vi "SeCrTs-RD Modified.vi"() -> ()   [LabVIEW 2022 SP3]
doc: "Datalog Redundant software"
uses:
  SeCrTS-Display And Datalog/Source Code/Control/SeCrTs-Enum.ctl
  Source Code/Globals/SeCrTs-RD globals.vi
panel:
  out "Logging?":bool
  out "Connected?":bool
  in  "Exit":bool
  out "Log Period(Min)":dbl
  out "Log type":bool
  in  "IP Address":string="169.254.222.222"
  out "error out":errorcluster
  # "DATALOG REDUNDANT SOFTWARE"
  # "VERSION           : V1.2\nRELEASE DATE : 23/09/2024"
  # "Periodical log"
  # "Continuous log"
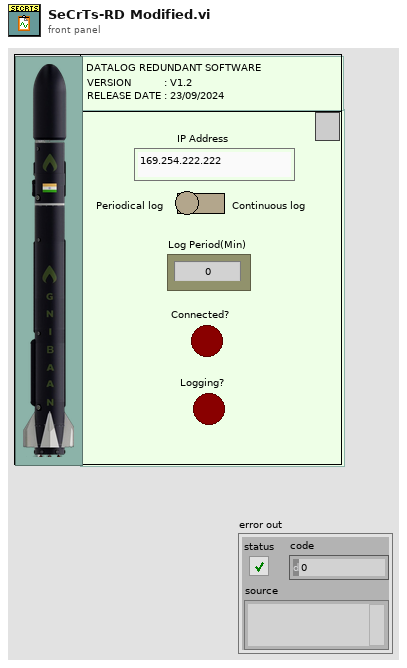
[diagram p1: front panel]
types:
  T1 = typedef "SeCrTs-Enum.ctl" = enum16{"Initialize", "Poll", "Establish ref", "Read", "Close", "Exit"}
  T2 = cluster{"Config":refnum<k21>, "log":refnum<k21>, "Log name":refnum<k21>, "C/NC":refnum<k21>, "Log time":refnum<k21>}
  T3 = enum8{"Enabled", "Disabled", "Disabled and Grayed Out"}
  T4 = cluster{"AO config":cluster{"Channel_Name":string, "Channel_Number":string, "Default_Value":dbl, "Units":string}[], "AI config":cluster{"Channel_Name":string, "Channel_Number":string, "Pre_Scale_min":dbl, "Pre_Scale_max":dbl, "Sensor_min":dbl, "Sensor_max":dbl, "Units":string}[], "DI config":cluster{"Channel_Name":string, "Channel_Number":string, "Default_Value":bool, "DI invert?":bool}[], "DO config":cluster{"Channel_Name":string, "Channel_Number":string, "Default_Value":bool, "DO invert?":bool}[], "TC config":cluster{"Channel_Name":string, "Channel_Number":string, "Pre_Scale_min":dbl, "Pre_Scale_max":dbl, "units":i32, " type":i32}[], "ACC config":cluster{"Channel_Name":string, "Channel_Number":string, "Pre_Scale_min":dbl, "Pre_Scale_max":dbl, "Terminal configuration":i32, "Sensitivity":dbl, "Sensitivity units":i32}[], "SG config":cluster{"Channel_Name":string, "Channel_Number":string, "Pre_Scale_min":dbl, "Pre_Scale_max":dbl}[], "Strain Gauge Settings":cluster{"poisson ratio":dbl, "nominal gage resistance":dbl, "gage factor":dbl}, "Bridge Settings":cluster{"voltage excitation value":dbl, "voltage excitation source":i32, "initial bridge voltage":dbl, "lead wire resistance":dbl, "strain configuration":i32}, "Sample Rate":cluster{"AI Sample Rate":dbl[], "AO Sample Rate":dbl[], "DI Sample Rate":dbl[], "TC Sample Rate":dbl[], "DO Sample Rate":dbl[], "SG Sample Rate":dbl[], "ACC Sample Rate":dbl[]}}
  T5 = enum32{"invalid app kind", "Development System", "Run Time System", "Student Edition", "Embedded LabVIEW", "Evaluation", "Custom"}
  T6 = cluster{"Datalog path":path, "Configuration path":path, "Signal list path":path, "Sub vi's":path, "Authentication":path}
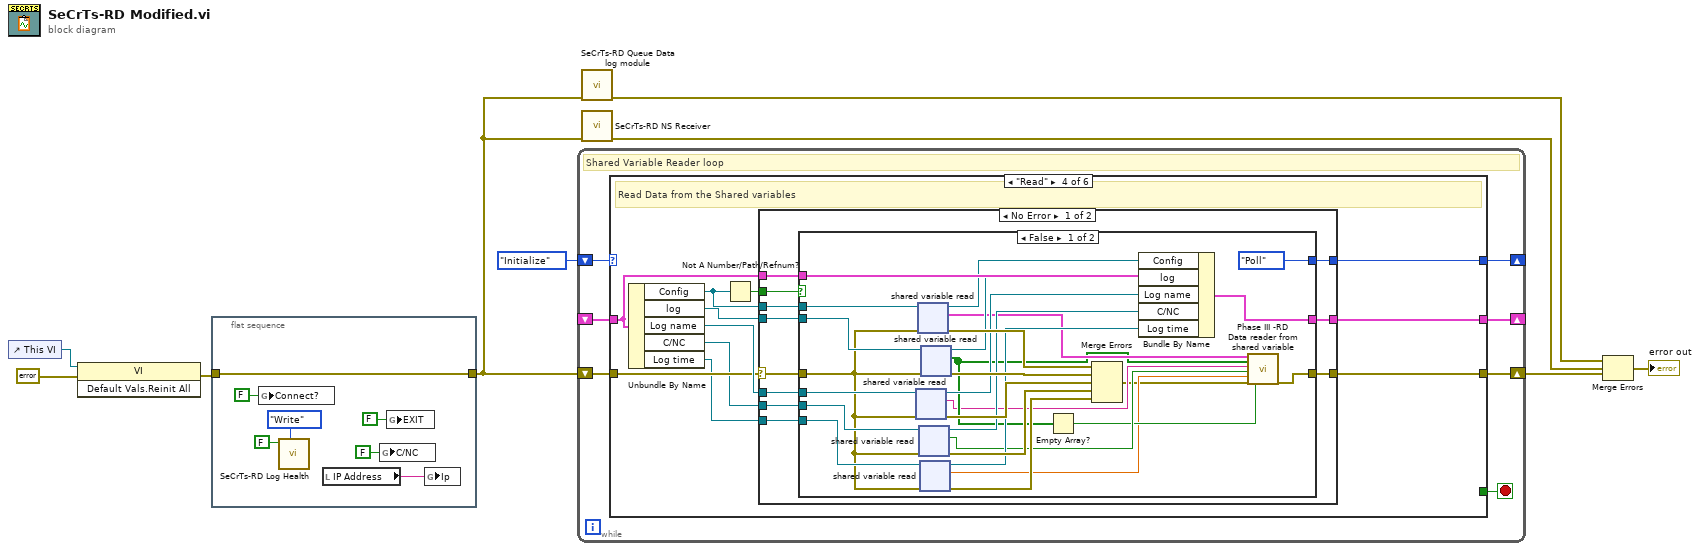
[diagram p0: block diagram]
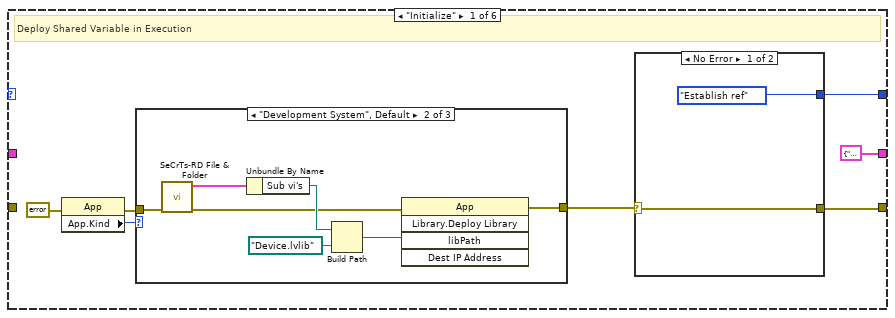
[diagram p2: hidden frame]
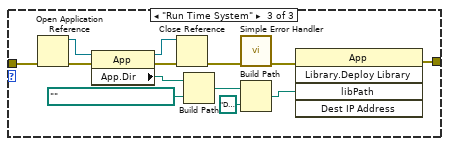
[diagram p4: hidden frame]
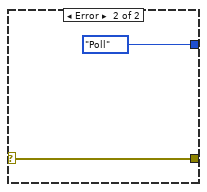
[diagram p5: hidden frame]
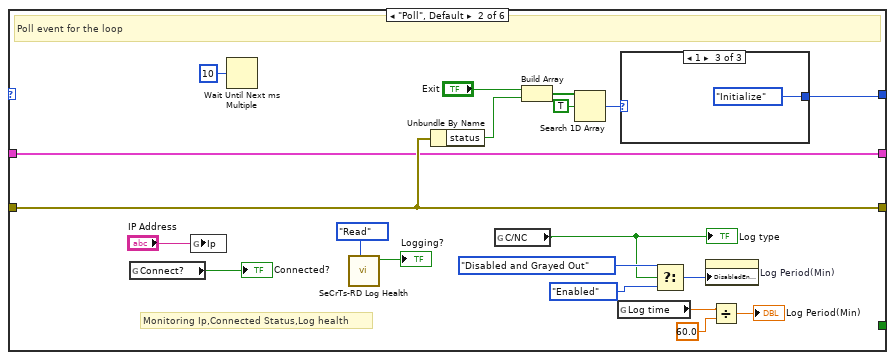
[diagram p6: hidden frame]
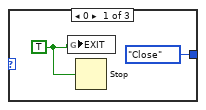
[diagram p7: hidden frame]
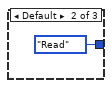
[diagram p8: hidden frame]
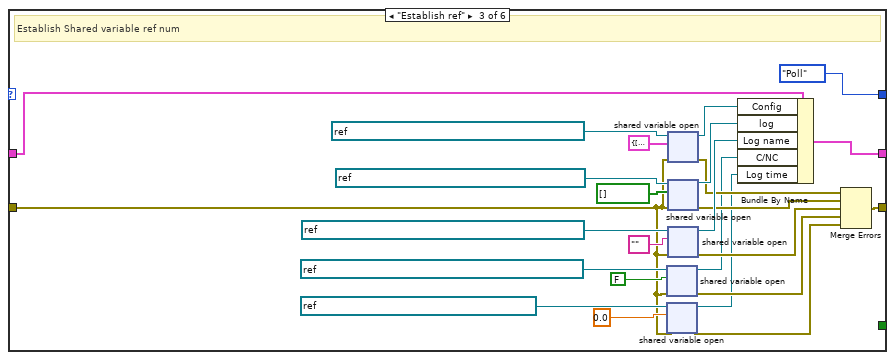
[diagram p9: hidden frame]
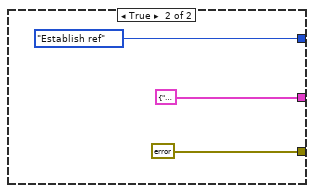
[diagram p10: hidden frame]
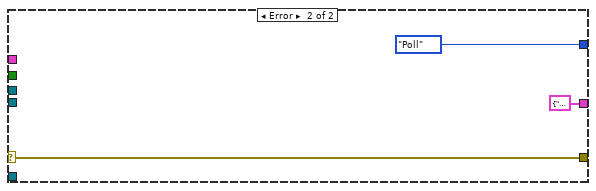
[diagram p11: hidden frame]
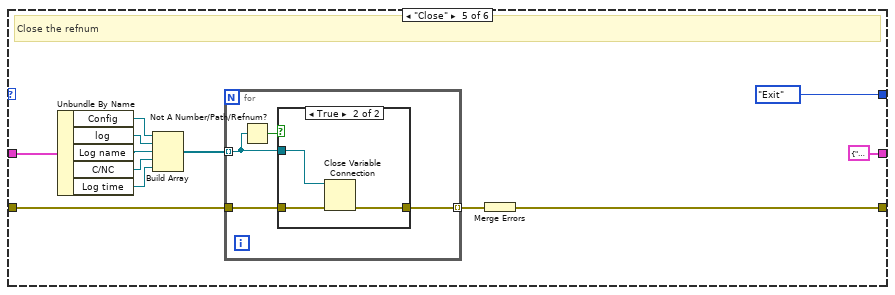
[diagram p12: hidden frame]
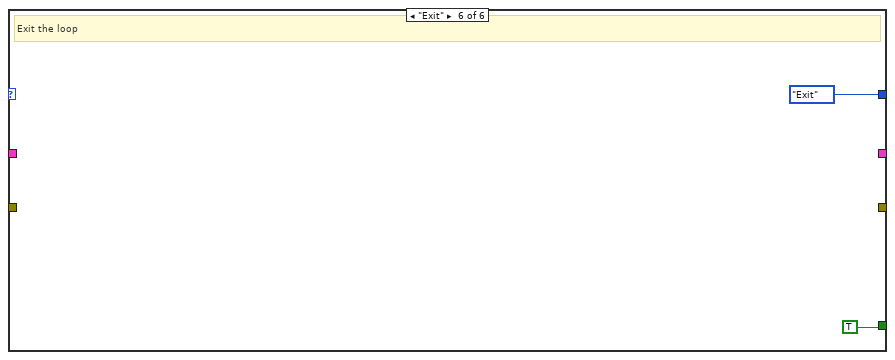
[diagram p14: hidden frame]
diagram:
  n1 = control-ref of="This VI"() -> (w3:refnum<vi>)
  n2 = invoke class="VI" method="Default Vals.Reinit All"(reference=w3, error in=errorcluster {"status"=FALSE, "code"=0, "source"=""} ("error in (no error)")) -> (error out=w2:errorcluster)  [unwired: 1 in, 2 out]
  n3 = flat-sequence {
    tunnel: w2 -> [w10]
    tunnel: [w10] -> w6
    frame #0 {
      n4 = global write "SeCrTs-RD globals.vi" "Connect?"(FALSE ("Connect?")) -> ()
      n5 = call "SeCrTs-RD Log Health.vi"("Enum"=enum16{"Read", "Write"}."Write", "Log health"=FALSE) -> ()  [unwired: 8 in, 2 out]
      n6 = local read "IP Address"() -> (w11:string)
      n7 = global write "SeCrTs-RD globals.vi" "C/NC"(FALSE ("C/NC")) -> ()
      n8 = global write "SeCrTs-RD globals.vi" "EXIT"(FALSE ("EXIT")) -> ()
      n9 = global write "SeCrTs-RD globals.vi" "Ip"(w11) -> ()
    }
  }
  n10 = while {
    shift-right: [w20] -> _
    shift-left: SeCrTs-Enum."Initialize" -> [w23]
    shift-right: [w21] -> w5
    shift-left: w6 -> [w22]
    shift-right: [w18] -> _
    shift-left: _ -> [w19]
    stop <- w17 stop-if-true
    # "Shared Variable Reader loop"
    n11 = case shown="\"Read\"" w23 {
      tunnel: w22 -> [_ w74 w84 w112 w166 _]
      tunnel: [w26 w74 w93 w107 w164 _] -> w21
      tunnel: [w30 w75 SeCrTs-Enum."Poll" w108 SeCrTs-Enum."Exit" SeCrTs-Enum."Exit"] -> w20
      tunnel: w19 -> [_ w69 w98 w110 w171 _]
      tunnel: [T2 {"Config"="", "log"="", "Log name"="", "C/NC"="", "Log time"=""} w69 w97 w109 T2 {"Config"="", "log"="", "Log name"="", "C/NC"="", "Log time"=""} _] -> w18
      tunnel: [_ _ _ _ _ TRUE] -> w17
      frame "Initialize" {
        # "Deploy Shared Variable in Execution"
        n12 = property class="App"(error in=errorcluster {"status"=FALSE, "code"=0, "source"=""} ("error out")) -> (error out=w24:errorcluster, "App.Kind"=w28:T5)  [unwired: 1 in, 1 out]
        n13 = case shown="\"Development System\", Default" w28 {
          tunnel: w24 -> [w31 w34 w42]
          tunnel: [w31 w35 w39] -> w27
          frame "invalid app kind" {
          }
          frame "Development System", Default {
            n14 = call "SeCrTs-RD File & Folder.vi"("error in (no error)"=w34) -> ("error out"=w32:errorcluster, "File Output"=w33:T6)  [unwired: 9 in]
            n15 = Unbundle By Name(w33) -> ("Sub vi's"=w37:path)
            n16 = Build Path(base path=w37, name or relative path=path "Device.lvlib") -> (appended path=w38:path)
            n17 = invoke class="App" method="Library.Deploy Library"(error in=w32, "libPath"=w38) -> (error out=w35:errorcluster)  [unwired: 3 in, 4 out]
          }
          frame "Run Time System" {
            n18 = Open Application Reference(8:w42) -> (0:w50:errorcluster, 3:w51:refnum<vi>)  [unwired: 3 in]
            n19 = property class="App"(reference=w51, error in=w50) -> (reference out=w48:refnum<vi>, error out=w49:errorcluster, "App.Dir"=w46:path)
            n20 = Close Reference(reference=w48, error in (no error)=w49) -> (error out=w47:errorcluster)
            n21 = Build Path(base path=w46, name or relative path=path "") -> (appended path=w45:path)
            n22 = call <vilib>:"Simple Error Handler.vi"("error in (no error)"=w47) -> ("error out"=w44:errorcluster)  [unwired: 4 in, 4 out]
            n23 = Build Path(base path=w45, name or relative path=path "Device.lvlib") -> (appended path=w43:path)
            n24 = invoke class="App" method="Library.Deploy Library"(error in=w44, "libPath"=w43) -> (error out=w39:errorcluster)  [unwired: 3 in, 4 out]
          }
        }
        n25 = case shown="No Error" w27 {
          selector: w27 -> [w52 w54]
          tunnel: [SeCrTs-Enum."Establish ref" SeCrTs-Enum."Poll"] -> w30
          tunnel: [w52 w54] -> w26
          frame No Error {
          }
          frame Error {
          }
        }
      }
      frame "Poll", Default {
        # "Monitoring Ip,Connected Status,Log health"
        # "Poll event for the loop"
        n26 = global read "SeCrTs-RD globals.vi" "Connect?"() -> (→"Connected?":bool)
        n27 = global write "SeCrTs-RD globals.vi" "Ip"("IP Address") -> ()
        n28 = Wait Until Next ms Multiple(millisecond multiple=u32 10) -> ()  [unwired: 1 out]
        n29 = call "SeCrTs-RD Log Health.vi"("Enum"=enum16{"Read", "Write"}."Read") -> ("Log health R"=→"Logging?":bool)  [unwired: 9 in, 1 out]
        n30 = Unbundle By Name(w74) -> ("status"=w73:bool)
        n31 = global read "SeCrTs-RD globals.vi" "C/NC"() -> (w59:bool)
        "Log type" <- w59
        n32 = Build Array("Exit", w73) -> (w71:bool[])
        n33 = Search 1D Array(1D array=w71, element=TRUE) -> (index of element=w72:i32)  [unwired: 1 in]
        n34 = global read "SeCrTs-RD globals.vi" "Log time"() -> (w58:dbl)
        n35 = case shown="1" w72 {
          tunnel: [SeCrTs-Enum."Close" SeCrTs-Enum."Read" SeCrTs-Enum."Initialize"] -> w75
          frame 0 {
            w76 = TRUE ("EXIT")
            n36 = global write "SeCrTs-RD globals.vi" "EXIT"(w76) -> ()
            n37 = Stop(stop? (T)=w76) -> ()
          }
          frame Default {
          }
          frame 1 {
          }
        }
        n38 = Select(t=T3."Disabled and Grayed Out" ("Disabled"), s=w59, f=T3."Enabled" ("Disabled")) -> (s? t:f=w64:T3)
        n39 = property on="Log Period(Min)" class="DigNum (strict)"("DisabledEnum"=w64) -> ()  [unwired: 2 in, 2 out]
        n40 = Divide(x=w58, y=60.0) -> (x/y=→"Log Period(Min)":dbl)
      }
      frame "Establish ref" {
        # "Establish Shared variable ref num"
        n41 = shared-variable-open(refnum<k21> "ni.var.psp://tto-pxie/Device/Continuous log%3F" ("shared variable refnum in"), w84, FALSE ("Continuous log?")) -> (w81:refnum<k21>, w83:errorcluster)  [unwired: 1 in]
        n42 = shared-variable-open(refnum<k21> "ni.var.psp://tto-pxie/Device/Log Period" ("shared variable refnum in"), w84, 0.0 ("Log Period")) -> (w80:refnum<k21>, w82:errorcluster)  [unwired: 1 in]
        n43 = shared-variable-open(refnum<k21> "ni.var.psp://tto-pxie/Device/Configuration" ("shared variable refnum in"), w84, T4 {"AO config"=[], "AI config"=[], "DI config"=[], "DO config"=[], "TC config"=[], "ACC config"=[], "SG config"=[], "Strain Gauge Settings"={"poisson ratio"=0.3, "nominal gage resistance"=120.0, "gage factor"=2.08}, "Bridge Settings"={"voltage excitation value"=3.3, "voltage excitation source"=10200, "initial bridge voltage"=0.0, "lead wire resistance"=1.7, "strain configuration"=10271}, "Sample Rate"={"AI Sample Rate"=[], "AO Sample Rate"=[], "DI Sample Rate"=[], "TC Sample Rate"=[], "DO Sample Rate"=[], "SG Sample Rate"=[], "ACC Sample Rate"=[]}} ("data")) -> (w96:refnum<k21>, w92:errorcluster)  [unwired: 1 in]
        n44 = shared-variable-open(refnum<k21> "ni.var.psp://tto-pxie/Device/Start Stop log" ("shared variable refnum in"), w84, bool[] [] ("Boolean")) -> (w95:refnum<k21>, w91:errorcluster)  [unwired: 1 in]
        n45 = shared-variable-open(refnum<k21> "ni.var.psp://tto-pxie/Device/Datalog phase code" ("shared variable refnum in"), w84, "") -> (w94:refnum<k21>, w90:errorcluster)  [unwired: 1 in]
        n46 = Bundle By Name(cluster=w98, "Config"=w96, "log"=w95, "Log name"=w94, "C/NC"=w81, "Log time"=w80) -> (w97:T2)
        n47 = Merge Errors(w92, w91, w90, w83, w82) -> (w93:errorcluster)
      }
      frame "Read" {
        # "Read Data from the Shared variables"
        n48 = Unbundle By Name(w110) -> ("Config"=w113:refnum<k21>, "log"=w115:refnum<k21>, "Log name"=w114:refnum<k21>, "C/NC"=w106:refnum<k21>, "Log time"=w105:refnum<k21>)
        n49 = Not A Number/Path/Refnum?(number/path/refnum=w113) -> (NaN/Path/Refnum?=w111:bool)
        n50 = case shown="No Error" w112 {
          selector: w112 -> [w122 w159]
          tunnel: w115 -> [w126 _]
          tunnel: w114 -> [w125 _]
          tunnel: w113 -> [w124 _]
          tunnel: w111 -> [w123 _]
          tunnel: w110 -> [w120 _]
          tunnel: [w119 T2 {"Config"="", "log"="", "Log name"="", "C/NC"="", "Log time"=""}] -> w109
          tunnel: [w118 SeCrTs-Enum."Poll"] -> w108
          tunnel: [w121 w159] -> w107
          tunnel: w106 -> [w117 _]
          tunnel: w105 -> [w116 _]
          frame No Error {
            n51 = case shown="False" w123 {
              tunnel: w126 -> [w153 _]
              tunnel: w125 -> [w152 _]
              tunnel: w124 -> [w151 _]
              tunnel: w122 -> [w138 _]
              tunnel: [w142 errorcluster {"status"=FALSE, "code"=0, "source"=""} ("error IO")] -> w121
              tunnel: w120 -> [w147 _]
              tunnel: [w146 T2 {"Config"="", "log"="", "Log name"="", "C/NC"="", "Log time"=""}] -> w119
              tunnel: [SeCrTs-Enum."Poll" SeCrTs-Enum."Establish ref"] -> w118
              tunnel: w117 -> [w140 _]
              tunnel: w116 -> [w139 _]
              frame False {
                n52 = shared-variable-read(w152, w138) -> (w143:refnum<k21>, w148:errorcluster, w131:string)  [unwired: 1 out]
                n53 = shared-variable-read(w151, w138) -> (w145:refnum<k21>, w150:errorcluster, w133:T4)  [unwired: 1 out]
                n54 = shared-variable-read(w140, w138) -> (w135:refnum<k21>, w137:errorcluster, w130:bool)  [unwired: 1 out]
                n55 = shared-variable-read(w139, w138) -> (w134:refnum<k21>, w136:errorcluster, w128:dbl)  [unwired: 1 out]
                n56 = shared-variable-read(w153, w138) -> (w144:refnum<k21>, w149:errorcluster, w132:bool[])  [unwired: 1 out]
                n57 = Empty Array?(array=w132) -> (empty?=w129:bool)
                n58 = Merge Errors(w150, w149, w148, w137, w136) -> (w127:errorcluster)
                n59 = Bundle By Name(cluster=w147, "Config"=w145, "log"=w144, "Log name"=w143, "C/NC"=w135, "Log time"=w134) -> (w146:T2)
                n60 = call "Phase III -RD Data reader from shared variable.vi"("Config"=w133, "Start/Stop Log"=w132, "Log Name"=w131, "C/NC"=w130, "Log min"=w128, "error IO"=w127, "empty?"=w129) -> ("error out"=w142:errorcluster)  [unwired: 12 in]
              }
              frame True {
              }
            }
          }
          frame Error {
          }
        }
      }
      frame "Close" {
        # "Close the refnum"
        n61 = Unbundle By Name(w171) -> ("Config"=w169:refnum<k21>, "log"=w168:refnum<k21>, "Log name"=w167:refnum<k21>, "C/NC"=w162:refnum<k21>, "Log time"=w161:refnum<k21>)
        n62 = Build Array(w169, w168, w167, w162, w161) -> (w170:refnum<k21>[])
        n63 = for {
          tunnel: w170 -> [w174] mode=indexing
          tunnel: w166 -> [w173]
          tunnel: [w172] -> w165 mode=indexing
          n64 = Not A Number/Path/Refnum?(number/path/refnum=w174) -> (NaN/Path/Refnum?=w175:bool)
          n65 = case shown="True" w175 {
            tunnel: w174 -> [_ w179]
            tunnel: w173 -> [w176 w178]
            tunnel: [w176 w177] -> w172
            frame False {
            }
            frame True {
              n66 = Close Variable Connection(8:w178, 11:w179) -> (0:w177:errorcluster)
            }
          }
        }
        n67 = Merge Errors(w165) -> (w164:errorcluster)
      }
      frame "Exit" {
        # "Exit the loop"
      }
    }
  }
  n68 = call "SeCrTs-RD Queue Data log module.vi"("error in"=w6) -> ("error out"=w9:errorcluster)  [unwired: 10 in]
  n69 = call "SeCrTs-RD NS Receiver.vi"("error in"=w6) -> ("error out"=w8:errorcluster)  [unwired: 10 in]
  n70 = Merge Errors(w9, w8, w5) -> (→"error out":errorcluster)
